vi "EnableDisable Main Page.vi"(8 "error in (no error)":errorcluster, 11 "Node Ptr":u64 format="%.0x") -> (0 "error out":errorcluster)   [LabVIEW 2015, in "Waveform-Processing-Custom-Device System Explorer.lvlib"]
uses:
  Waveform-Processing-Custom-Device System Explorer.lvlib
  Shared/Constants.vi
  <vilib>/NI VeriStand/Custom Device API/Custom Device API.lvlib
  Shared/Waveform-Processing-Custom-Device Shared.lvlib
panel:
  in  "Tag":string
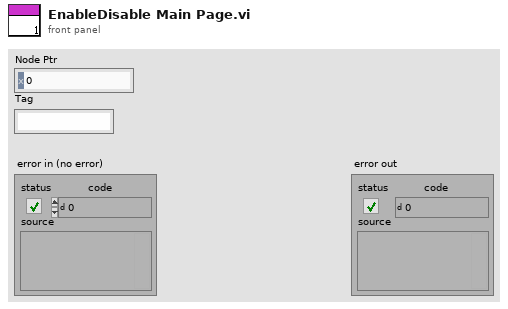
[diagram p1: front panel]
types:
  T1 = typedef "Custom Device API.lvlib/Custom Device Item Ref.ctl" = u64
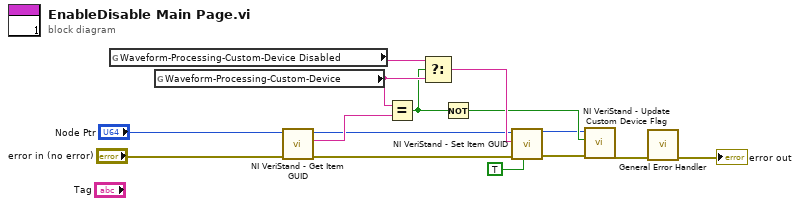
[diagram p0: block diagram]
diagram:
  n1 = global read "Constants.vi" "Waveform-Processing-Custom-Device Disabled"() -> (w12:string)
  n2 = global read "Constants.vi" "Waveform-Processing-Custom-Device"() -> (w11:string)
  n3 = call <vilib>:"NI VeriStand - Get Item GUID.vi"("error in (no error)"="error in (no error)", "Item Ref in"="Node Ptr") -> ("error out"=w7:errorcluster, "GUID"=w14:string, "Item Ref out"=w8:T1)  [unwired: 7 in]
  n4 = Equal?(x=w11, y=w14) -> (x = y?=w10:bool)
  n5 = Select(t=w12, s=w10, f=w11) -> (s? t:f=w9:string)
  n6 = Not(x=w10) -> (.not. x?=w5:bool)
  n7 = call <vilib>:"NI VeriStand - Set Item GUID.vi"("Refresh System Explorer Tree? (F)"=TRUE, "error in (no error)"=w7, "GUID"=w9, "Item Ref in"=w8) -> ("error out"=w6:errorcluster, "Item Ref out"=w4:T1)  [unwired: 6 in]
  n8 = call <vilib>:"NI VeriStand - Update Custom Device Flag.vi"("error in (no error)"=w6, "Is Custom Device Active?"=w5, "Device Ref in"=w4) -> ("error out"=w3:errorcluster)  [unwired: 7 in, 1 out]
  n9 = call <vilib>:"General Error Handler.vi"("error in (no error)"=w3) -> ("error out"=→"error out":errorcluster)  [unwired: 10 in, 4 out]
